vi "MetaLaunchPythonServer.vi"(11 "Compiler Settings":T1={"Python Path"=path "", "Main File"="mainscript.py", "Meta File"="metascript.txt", "Aux File"="auxscript.py", "Pre File"="metascript.txt"}) -> ()   [LabVIEW 2019]
uses:
  PulseCompiler/CompilerSettings.ctl
panel:
  out "standard error":string
  out "standard output":string
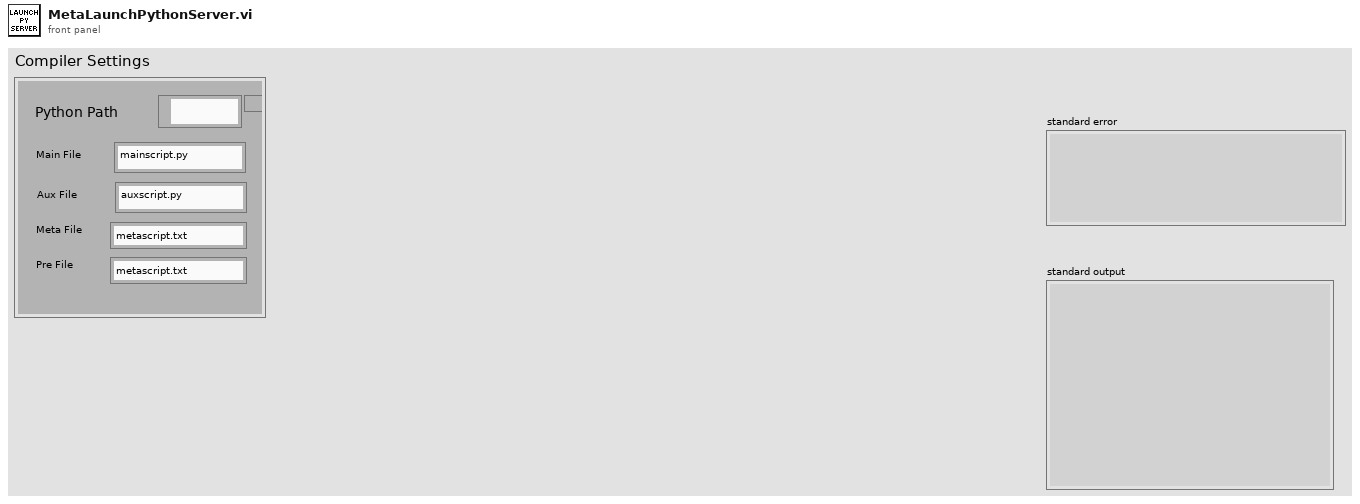
[diagram p1: front panel]
types:
  T1 = typedef "CompilerSettings.ctl" = cluster{"Python Path":path, "Main File":string, "Meta File":string, "Aux File":string, "Pre File":string}
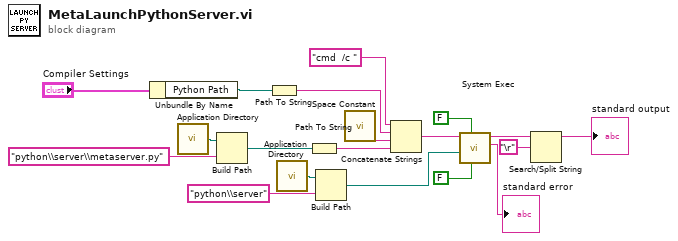
[diagram p0: block diagram]
diagram:
  n1 = Unbundle By Name("Compiler Settings") -> ("Python Path"=w2:path)
  n2 = call <vilib>:"Application Directory.vi"() -> ("Application Directory"=w14:path)
  n3 = Build Path(base path=w14, name or relative path="python\\server\\metaserver.py") -> (appended path=w16:path)
  n4 = Path To String(path=w2) -> (string=w1:string)
  n5 = call <vilib>:"Application Directory.vi"() -> ("Application Directory"=w7:path)
  n6 = Path To String(path=w16) -> (string=w17:string)
  n7 = Build Path(base path=w7, name or relative path="python\\server") -> (appended path=w9:path)
  n8 = call <vilib>:"Space Constant.vi"() -> ("String"=w13:string)
  n9 = Concatenate Strings("cmd  /c " ("string"), w1, w13, w17) -> (w3:string)
  n10 = call <vilib>:"System Exec.vi"("run minimized? (F)"=FALSE, "wait until completion? (T)"=FALSE, "working directory"=w9, "command line"=w3) -> ("standard error"=→"standard error":string, "standard output"=w5:string)  [unwired: 4 in, 2 out]
  n11 = Search/Split String(string=w5, search string/char (-)="\r") -> (substring before match=→"standard output":string)  [unwired: 1 in, 2 out]
